vi "AI.vi"(6 "external shunt resistor value":dbl=1.0 format="%#_13g", 7 "Mode":enum16{"Voltage", "Current"}(ring), 8 "error in":errorcluster caption="错误输入", 10 "Channel":string(combo)="AI0", 11 "DAQmx设备名":tag="Dev7") -> (0 "error out":errorcluster caption="错误输出", 3 "data":dbl format="%.4f")   [LabVIEW 2013]
uses:
  <vilib>/DAQmx/read.llb/DAQmx Read (Analog DBL 1Chan 1Samp).vi
  <vilib>/DAQmx/create/channels.llb/DAQmx Create Channel (AI-Voltage-Basic).vi
  <vilib>/DAQmx/create/channels.llb/DAQmx Create Channel (AI-Current-Basic).vi
  <vilib>/DAQmx/miscellaneous.llb/DAQmx Fill In Error Info.vi
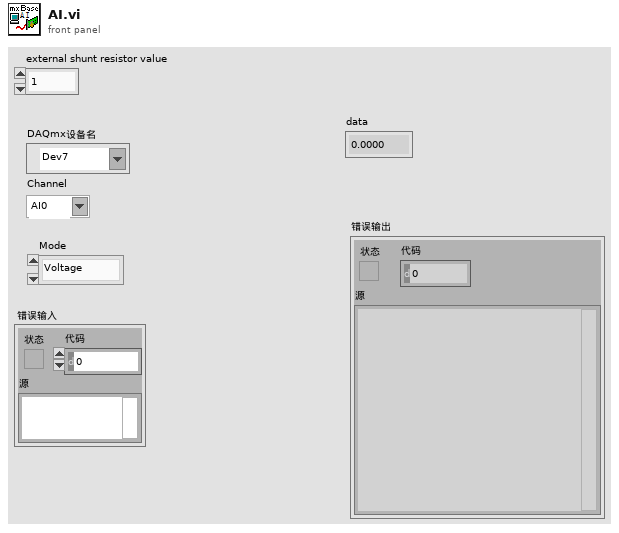
[diagram p1: front panel]
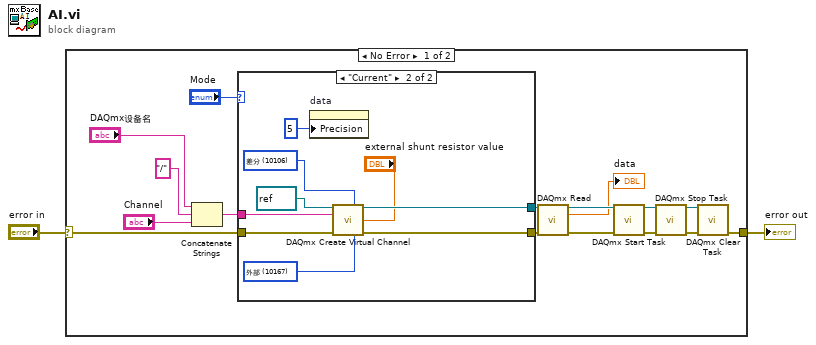
[diagram p0: block diagram]
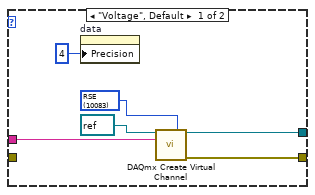
[diagram p2: hidden frame]
diagram:
  n1 = case shown="No Error" "error in" {
    selector: "error in" -> [w3 w34]
    tunnel: [w9 w34] -> w2
    frame No Error {
      n2 = Concatenate Strings("DAQmx设备名", "/" ("字符串"), "Channel") -> (w8:string)
      n3 = case shown="\"Current\"" "Mode" {
        tunnel: [w24 w33] -> w16
        tunnel: w8 -> [w22 w32]
        tunnel: [w20 w30] -> w7
        tunnel: w3 -> [_ w25]
        frame "Voltage", Default {
          w21 = 10083 items=["默认"=-1, "RSE"=10083, "NRSE"=10078, "差分"=10106, "伪差分"=12529] ("input terminal configuration")
          n4 = property on="data" class="DigNum (strict)"("Precision"=u8 4 ("显示格式:精度")) -> ()  [unwired: 2 in, 2 out]
          n5 = call-poly <vilib>:"DAQmx Create Virtual Channel.vi"("task in"=refnum<k21> refnum, "input terminal configuration"=w21, "physical channels"=w22) -> ("task out"=w24:refnum<k21>, "error out"=w20:errorcluster)  [unwired: 11 in]
        }
        frame "Current" {
          w28 = 10167 items=["默认"=-1, "内部"=10200, "外部"=10167] ("shunt resistor location")
          w29 = 10106 items=["默认"=-1, "RSE"=10083, "NRSE"=10078, "差分"=10106, "伪差分"=12529] ("input terminal configuration")
          n6 = property on="data" class="DigNum (strict)"("Precision"=u8 5 ("显示格式:精度")) -> ()  [unwired: 2 in, 2 out]
          n7 = call-poly <vilib>:"DAQmx Create Virtual Channel.vi"("task in"=refnum<k21> refnum, "input terminal configuration"=w29, "physical channels"=w32, "external shunt resistor value"="external shunt resistor value", "error in"=w25, "shunt resistor location"=w28) -> ("task out"=w33:refnum<k21>, "error out"=w30:errorcluster)  [unwired: 8 in]
        }
      }
      n8 = call-poly <vilib>:"DAQmx Read.vi"("task/channels in"=w16, "error in"=w7) -> ("task out"=w14:refnum<k21>, "data"=→"data":dbl, "error out"=w6:errorcluster)  [unwired: 11 in]
      n9 = call <vilib>:"DAQmx Start Task.vi"("task/channels in"=w14, "error in"=w6) -> ("task out"=w13:refnum<k21>, "error out"=w12:errorcluster)  [unwired: 12 in]
      n10 = call <vilib>:"DAQmx Stop Task.vi"("task/channels in"=w13, "error in"=w12) -> ("task out"=w11:refnum<k21>, "error out"=w10:errorcluster)  [unwired: 12 in]
      n11 = call <vilib>:"DAQmx Clear Task.vi"("task in"=w11, "error in"=w10) -> ("error out"=w9:errorcluster)  [unwired: 13 in]
    }
    frame Error {
    }
  }
  "error out" <- w2
